vi "7_Stream Sequence Low Level API.vi"() -> ()   [LabVIEW 2014]
uses:
  <vilib>/Swabian Instruments/Pulse Streamer/PulseStreamer/PulseStreamer/typedefs/typedef_TriggerStart.ctl
  <vilib>/Swabian Instruments/Pulse Streamer/PulseStreamer/compat/typedef_Pulse.ctl
  <vilib>/Swabian Instruments/Pulse Streamer/PulseStreamer/PulseStreamer/stream/stream (Pulses).vi
  <vilib>/Swabian Instruments/Pulse Streamer/PulseStreamer/PulseStreamer/PulseStreamer.lvclass
  <vilib>/Swabian Instruments/Pulse Streamer/PulseStreamer/PulseStreamer.lvlib
panel:
  in  "Final state":T1 {"digi mask" format="%b"}
  in  "Raw pulse sequence":T1[](array[typedef])=[{"duration"=1000, "digi mask"=255, "a0 (V)"=1.0, "a1 (V)"=-1.0}, {"duration"=100, "digi mask"=192, "a0 (V)"=0.800000011920929, "a1 (V)"=-0.800000011920929}, {"duration"=100, "digi mask"=48, "a0 (V)"=0.6000000238418579, "a1 (V)"=-0.6000000238418579}, {"duration"=100, "digi mask"=12, "a0 (V)"=0.4000000059604645, "a1 (V)"=-0.4000000059604645}, {"duration"=100, "digi mask"=3, "a0 (V)"=0.20000000298023224, "a1 (V)"=-0.20000000298023224}, {"duration"=1000, "digi mask"=0, "a0 (V)"=0.0, "a1 (V)"=0.0}] {"digi mask" format="%b"}
  in  "Initial Digital":bool[](array[boolean])=[FALSE, FALSE, FALSE, FALSE, FALSE, FALSE, FALSE, FALSE]
  in  "ip or hostname":string="pulsestreamer"
  in  "nRuns":i64=1
  out "error out":errorcluster
  in  "Init Analog 1  [V]":dbl min=-1.0 max=1.0 step=0.001
  in  "Init Analog 0 [V]":dbl min=-1.0 max=1.0 step=0.001
  in  "Start Type":T2
  # "repeat sequence nRuns time (if nRuns <0 then infinte loop)"
  # "Defines whether the sequence starts \n* immediatly after it was uploaded  (IMMEDIATE)\n* after a software trigger (startNow) has been sent (SOFTWARE)\n* with an external trigger signal to \"Trigger\" input on the corresponding edge (HW_RISING, HW_FALLING, HW_BOTH)."
  # "This is the binary representation of the sequence.\nThe digital output state is a 8 bit unsigned integer (each bit corresponds to high/low an output channel.\nThe analog is a 16 bit signed integer. The maximum value (32767) corresponds to +1V and the minimum value (-32768) to -1V.\n\nThis is the most direct way to program a sequence. The more comfortable way is shown in the next example."
  # "Initial State before generating the sequence\nIt is only important when\nStart Type <-> Immediate."
  # "Important remark: \nThe total duration of a single sequence (without the repetition) must be a multiple of 8 ns. \nFor durations which are not multiples of 8 ns the end of the sequence is padded with the very same value until a multiple of 8 ns is reached.\nExample:\nA sequence with duration 100 ns will be 104 ns because 12.5 * 8 ns = 100 ns, which will be padded to 13 * 8 ns = 104 ns."
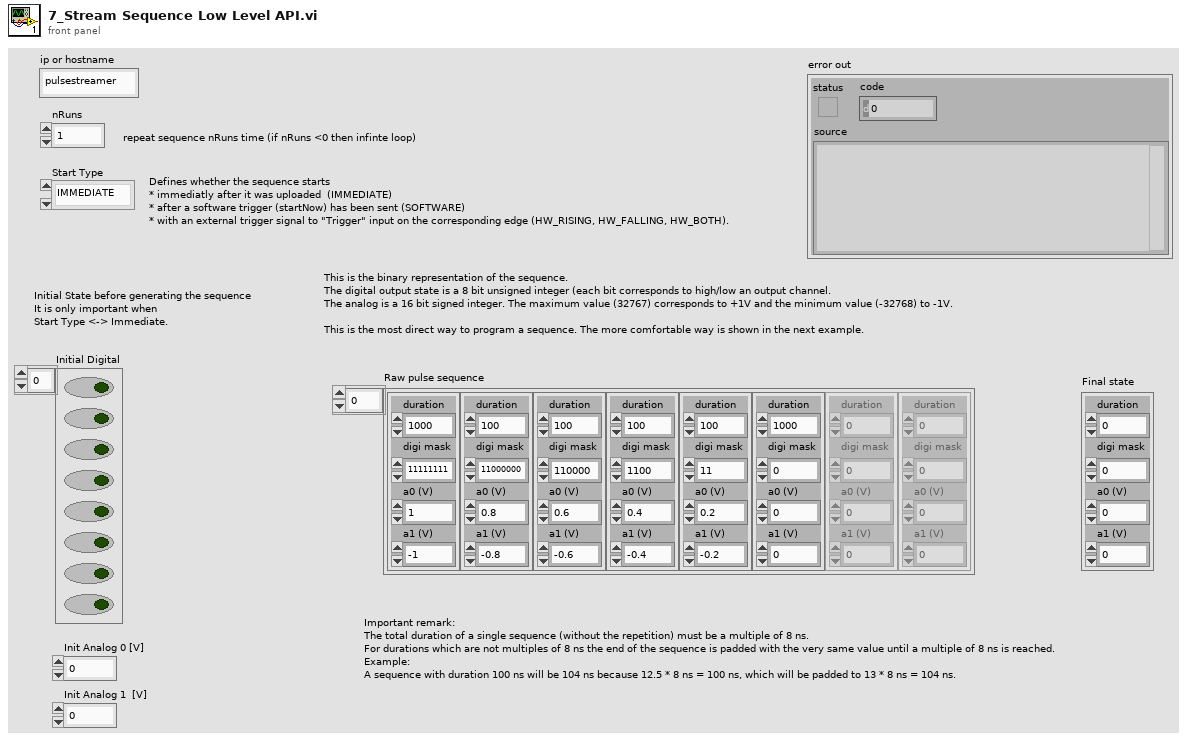
[diagram p1: front panel]
types:
  T1 = typedef "PulseStreamer.lvlib/typedef_Pulse.ctl" = cluster{"duration":i64, "digi mask":u8, "a0 (V)":dbl, "a1 (V)":dbl}
  T2 = typedef "PulseStreamer.lvlib/PulseStreamer.lvclass/typedef_TriggerStart.ctl" = enum16{"IMMEDIATE", "SOFTWARE", "HW_RISING", "HW_FALLING", "HW_RISING_AND_FALLING"}
  T3 = typedef "PulseStreamer.lvlib/typedef_OutputState.ctl" = cluster{"channels":T4[], "a0":dbl, "a1":dbl}
  T4 = typedef "PulseStreamer.lvlib/typedef_ChannelNumber.ctl" = i16
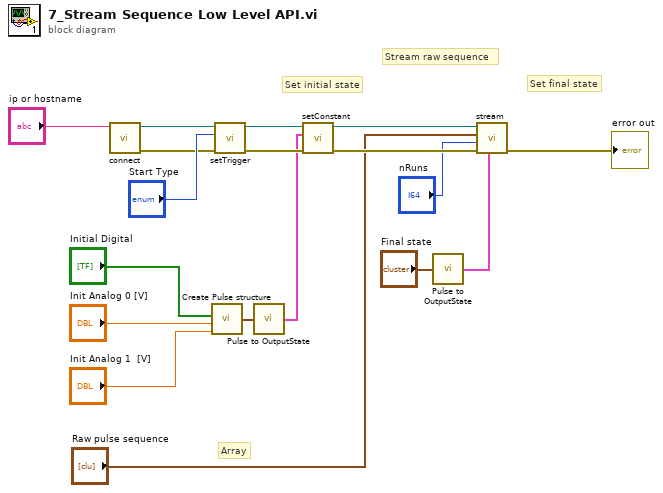
[diagram p0: block diagram]
diagram:
  # "Array"
  # "Stream raw sequence"
  # "Set final state"
  # "Set initial state"
  n1 = call <vilib>:"connect.vi"("ip"="ip or hostname") -> ("error out"=w16:errorcluster, "Pulse Streamer out"=w15:refnum<class "PulseStreamer.lvclass">)  [unwired: 9 in]
  n2 = call <vilib>:"Create Pulse structure.vi"("Analog 1"="Init Analog 1  [V]", "Analog 0"="Init Analog 0 [V]", "Digital"="Initial Digital") -> ("Pulse"=w2:T1)  [unwired: 1 in]
  n3 = call-dynamic "setTrigger.vi"("error in (no error)"=w16, "start"="Start Type", "Pulse Streamer in"=w15) -> ("error out"=w11:errorcluster, "Pulse Streamer out"=w10:refnum<class "PulseStreamer.lvclass">)  [unwired: 7 in]
  n4 = call <vilib>:"Pulse to OutputState.vi"("Pulse"=w2) -> ("OutputState"=w1:T3)
  n5 = call-dynamic "setConstant.vi"("error in (no error)"=w11, "outputState"=w1, "Pulse Streamer in"=w10) -> ("error out"=w8:errorcluster, "Pulse Streamer out"=w9:refnum<class "PulseStreamer.lvclass">)  [unwired: 7 in]
  n6 = call <vilib>:"Pulse to OutputState.vi"("Pulse"="Final state") -> ("OutputState"=w4:T3)
  n7 = call-poly <vilib>:"stream.vi"("Final state"=w4, "error in (no error)"=w8, "nRuns"="nRuns", "pulses"="Raw pulse sequence", "Pulse Streamer in"=w9) -> ("error out"=→"error out":errorcluster)  [unwired: 3 in, 1 out]
